vi "GNSS1-SET-3.vi"(4 "引用":refnum<vi>, 5 "Enum引用句柄":refnum<vi>, 6 "AbsTime引用句柄":refnum<vi>, 7 "Ring引用句柄":refnum<vi>, 8 "DigNum引用句柄":refnum<vi>, 9 "Enum引用句柄 2":refnum<vi>, 10 "DigNum引用句柄 2":refnum<vi>, 11 "Digital输入":refnum<vi>) -> (3 "添加的数组3":u8[](array[numeric]))   [LabVIEW 2012]
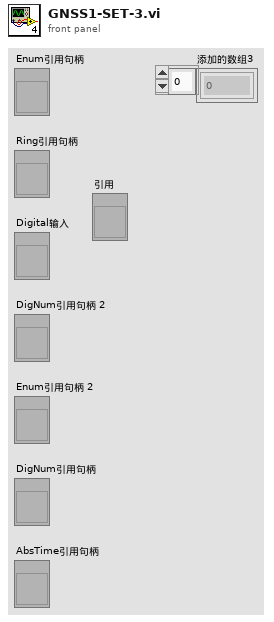
[diagram p1: front panel]
types:
  T1 = cluster{"BD北向速度":sgl, "BD东向速度":sgl, "BD天向速度":sgl, "BD经度":sgl, "BD纬度":sgl, "BD高度":sgl}
  T2 = typedef "LVDateTimeRec.ctl" = cluster{"秒数的小数部分":dbl, "秒":i32, "分":i32, "时":i32, "日":i32, "月":i32, "年":i32, "天数（周）":i32, "天数（年）":i32, "DST":i32}
  T3 = enum8{"无故障", "未正常初始化", "PDOP值>12", "没有可用卫星", "只有1颗可用卫星", "只有2颗可用卫星", "只有3颗可用卫星", "观测矩阵不可求逆", "定位解算不收敛", "高程超差", "速度大于10km/s"}
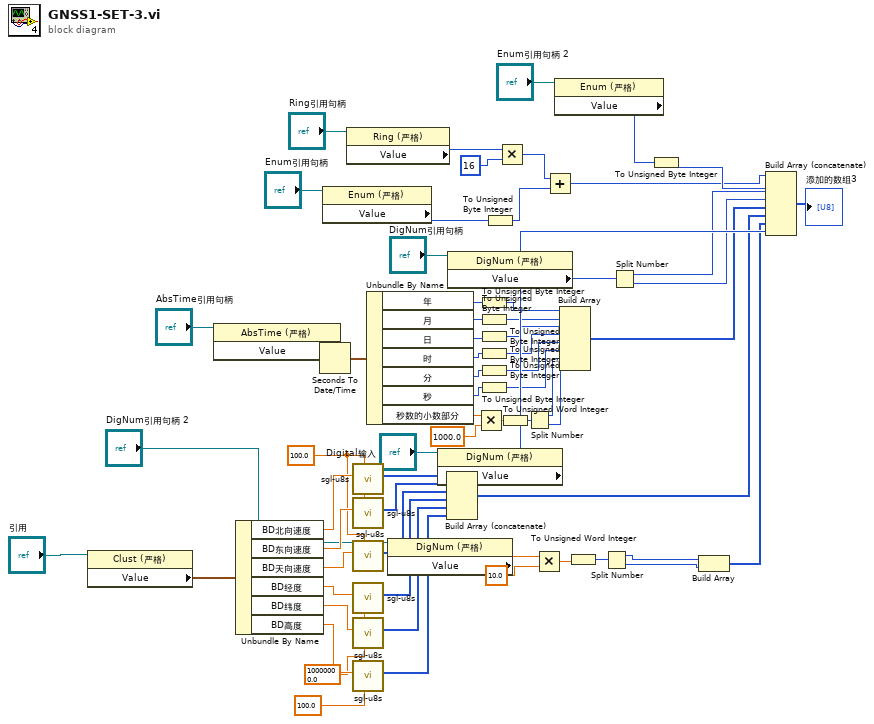
[diagram p0: block diagram]
diagram:
  w10 = sgl 10000000.0 ("精度")
  w23 = sgl 100.0 ("y")
  n1 = property on="属性节点" class="Clust (严格)"(reference="引用") -> ("Value"=w63:T1)  [unwired: 1 in, 2 out]
  n2 = property on="属性节点" class="AbsTime (严格)"(reference="AbsTime引用句柄") -> ("Value"=w62:timestamp)  [unwired: 1 in, 2 out]
  n3 = Unbundle By Name(w63) -> ("BD北向速度"=w30:sgl, "BD东向速度"=w28:sgl, "BD天向速度"=w27:sgl, "BD经度"=w26:sgl, "BD纬度"=w25:sgl, "BD高度"=w24:sgl)
  n4 = Seconds To Date/Time(time stamp (now)=w62) -> (date time rec=w50:T2)  [unwired: 1 in]
  n5 = property on="属性节点" class="Enum (严格)"(reference="Enum引用句柄") -> ("Value"=w56:T3)  [unwired: 1 in, 2 out]
  n6 = property on="属性节点" class="Ring (严格)"(reference="Ring引用句柄") -> ("Value"=w57:u8)  [unwired: 1 in, 2 out]
  n7 = call "sgl-u8s.vi"("输入sgl"=w30, "精度"=w23) -> ("u8s"=w29:u8[])  [unwired: 8 in]
  n8 = call "sgl-u8s.vi"("输入sgl"=w28, "精度"=w23) -> ("u8s"=w22:u8[])  [unwired: 8 in]
  n9 = call "sgl-u8s.vi"("输入sgl"=w27, "精度"=w23) -> ("u8s"=w21:u8[])  [unwired: 8 in]
  n10 = call "sgl-u8s.vi"("输入sgl"=w26, "精度"=w10) -> ("u8s"=w20:u8[])  [unwired: 8 in]
  n11 = call "sgl-u8s.vi"("输入sgl"=w25, "精度"=w10) -> ("u8s"=w19:u8[])  [unwired: 8 in]
  n12 = call "sgl-u8s.vi"("输入sgl"=w24, "精度"=sgl 100.0) -> ("u8s"=w18:u8[])  [unwired: 8 in]
  n13 = Unbundle By Name(w50) -> ("年"=w49:i32, "月"=w47:i32, "日"=w46:i32, "时"=w45:i32, "分"=w44:i32, "秒"=w43:i32, "秒数的小数部分"=w42:dbl)
  n14 = property on="属性节点" class="DigNum (严格)"(reference="DigNum引用句柄 2") -> ("Value"=w64:sgl)  [unwired: 1 in, 2 out]
  n15 = property on="属性节点" class="DigNum (严格)"(reference="Digital输入") -> ("Value"=w65:u8)  [unwired: 1 in, 2 out]
  n16 = Build Array (concatenate)(w29, w22, w21, w20, w19, w18) -> (w17:u8[])
  n17 = property on="属性节点" class="DigNum (严格)"(reference="DigNum引用句柄") -> ("Value"=w61:u16)  [unwired: 1 in, 2 out]
  n18 = Multiply(x=w42, y=1000.0) -> (x*y=w40:dbl)
  n19 = To Unsigned Byte Integer(number=w49) -> (unsigned 8bit integer=w48:u8)
  n20 = To Unsigned Byte Integer(number=w47) -> (unsigned 8bit integer=w38:u8)
  n21 = To Unsigned Byte Integer(number=w46) -> (unsigned 8bit integer=w37:u8)
  n22 = To Unsigned Byte Integer(number=w45) -> (unsigned 8bit integer=w36:u8)
  n23 = To Unsigned Byte Integer(number=w44) -> (unsigned 8bit integer=w35:u8)
  n24 = To Unsigned Byte Integer(number=w43) -> (unsigned 8bit integer=w34:u8)
  n25 = To Unsigned Byte Integer(number=w56) -> (unsigned 8bit integer=w53:u8)
  n26 = Multiply(x=w57, y=u8 16) -> (x*y=w54:u8)
  n27 = To Unsigned Word Integer(number=w40) -> (unsigned 16bit integer=w39:u16)
  n28 = Split Number(x=w39) -> (hi(x)=w33:u8, lo(x)=w32:u8)
  n29 = Multiply(x=w64, y=sgl 10.0) -> (x*y=w15:sgl)
  n30 = Add(x=w54, y=w53) -> (x+y=w59:u8)
  n31 = property on="属性节点" class="Enum (严格)"(reference="Enum引用句柄 2") -> ("Value"=w58:enum8{"无效", "定点定位", "差分定位"})  [unwired: 1 in, 2 out]
  n32 = Build Array(w48, w38, w37, w36, w35, w34, w33, w32) -> (w31:u8[])
  n33 = To Unsigned Word Integer(number=w15) -> (unsigned 16bit integer=w12:u16)
  n34 = Split Number(x=w12) -> (hi(x)=w14:u8, lo(x)=w13:u8)
  n35 = Split Number(x=w61) -> (hi(x)=w52:u8, lo(x)=w51:u8)
  n36 = To Unsigned Byte Integer(number=w58) -> (unsigned 8bit integer=w60:u8)
  n37 = Build Array(w14, w13) -> (w11:u8[])
  n38 = Build Array (concatenate)(w59, w60, w52, w51, w31, w17, w11, w65) -> (→"添加的数组3":u8[])
